vi "ABB Calc efficiency2.vi"(0 "Rated Data":T3, 1 "max wdg rise":dbl, 2 "Stator wdg":enum16{"Star", "Delta"}(ring), 3 "Stator  Phase resistance":dbl, 5 "Ambient temp":dbl, 7 "Frequency (Hz)":dbl, 9 "Efficiency Standard":enum16{"IEC 60034", "NEMA", "IEC 61972"}(ring), 11 "Specified  Power Factor":dbl[](array[numeric]), 12 "Selected Loads (% Rated)":dbl[](array[numeric]), 13 "Ohms":cluster{"Stator":dbl[], "Rotor":dbl[]}, 14 "Losses at rated voltage":T2, 15 "slip entry":T1={"Slip Source"=enum."Calculated", "Slip Entry"=[0.0, 0.0, 0.0, 0.0]}) -> (4 "Efficiency out":dbl[][](array[numeric]), 6 "Effy Temp":dbl, 8 "R at EffyT":cluster{"Stator":dbl[], "Rotor":dbl[]})   [LabVIEW 2017]
panel:
  out "mech+Iron":dbl
  # "Calculated slip"
  # "Mechanical Loss  (kW)"
  # "Iron Loss (kW)"
  # "Stator Copper Loss (kW)"
  # "Rotor Copper Loss (kW)"
  # "Stray load loss (kW)"
  # "Total loss (kW)"
  # "Load (kW)"
  # "Efficiency (%)"
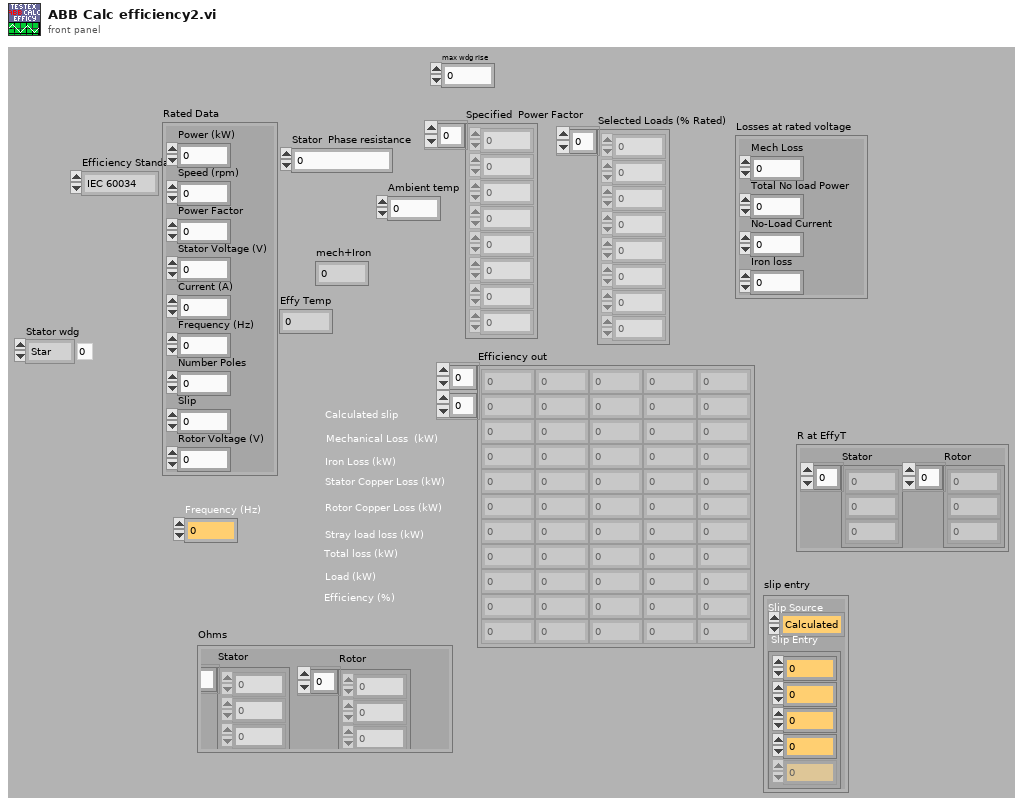
[diagram p1: front panel]
types:
  T1 = cluster{"Slip Source":enum16{"Calculated", "Entered"}, "Slip Entry":dbl[]}
  T2 = cluster{"Mech Loss":dbl, "Total No load Power":dbl, "No-Load Current":dbl, "Iron loss":dbl}
  T3 = cluster{"Power (kW)":dbl, "Speed (rpm)":dbl, "Power Factor":dbl, "Stator Voltage (V)":dbl, "Current (A)":dbl, "Frequency (Hz)":dbl, "Number Poles":dbl, "Slip":dbl, "Rotor Voltage (V)":dbl}
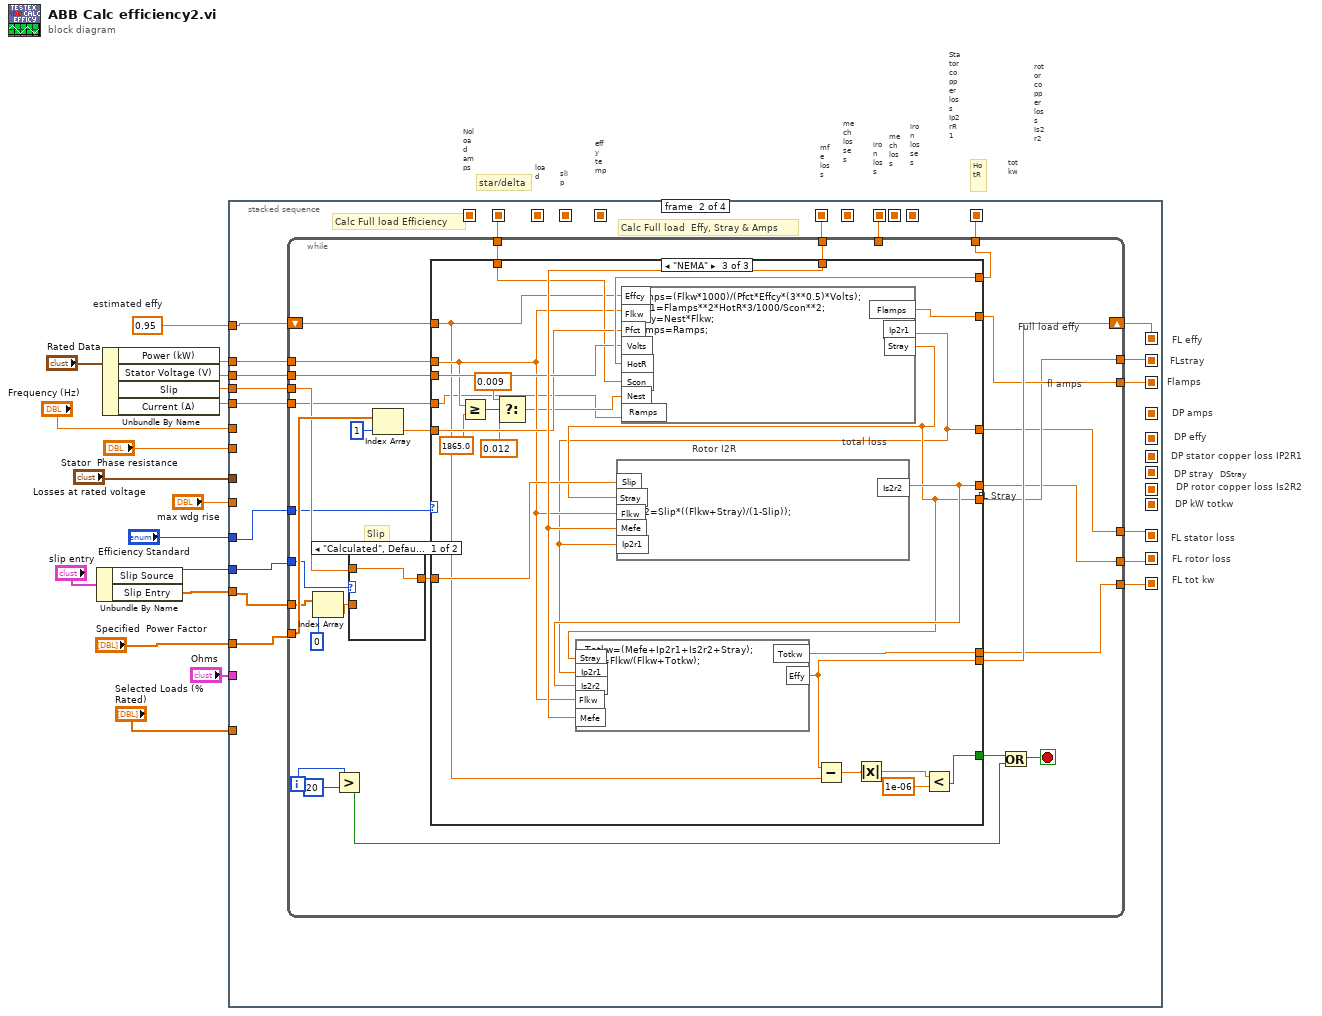
[diagram p0: block diagram]
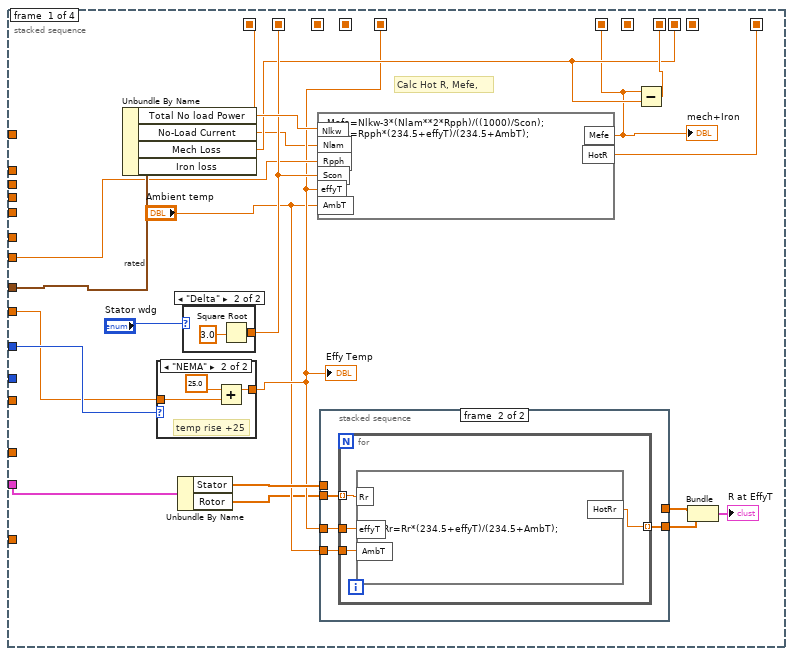
[diagram p2: hidden frame]
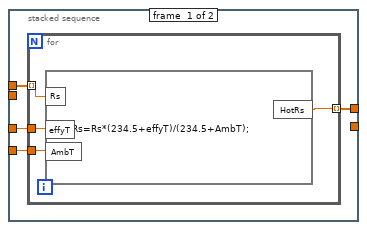
[diagram p3: hidden frame]
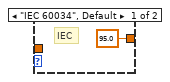
[diagram p4: hidden frame]
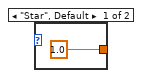
[diagram p5: hidden frame]
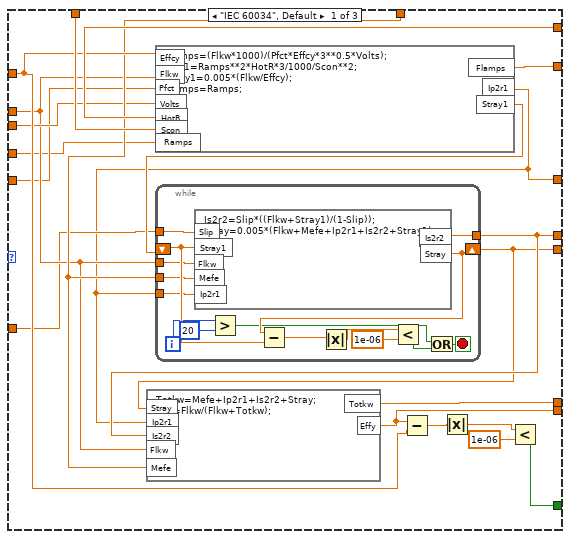
[diagram p6: hidden frame]
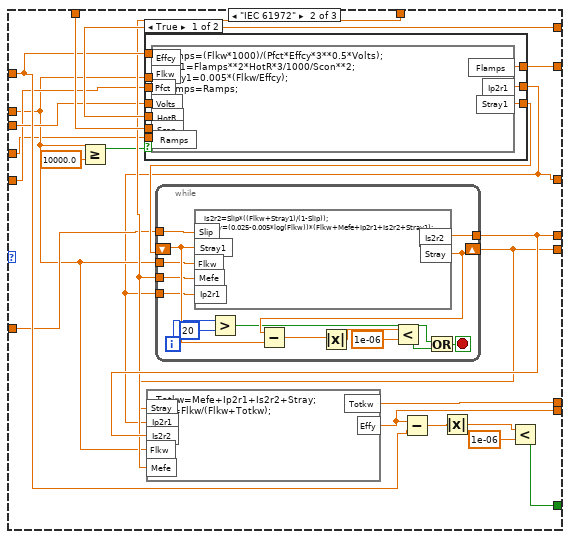
[diagram p7: hidden frame]
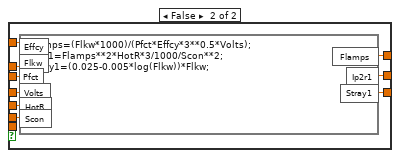
[diagram p8: hidden frame]
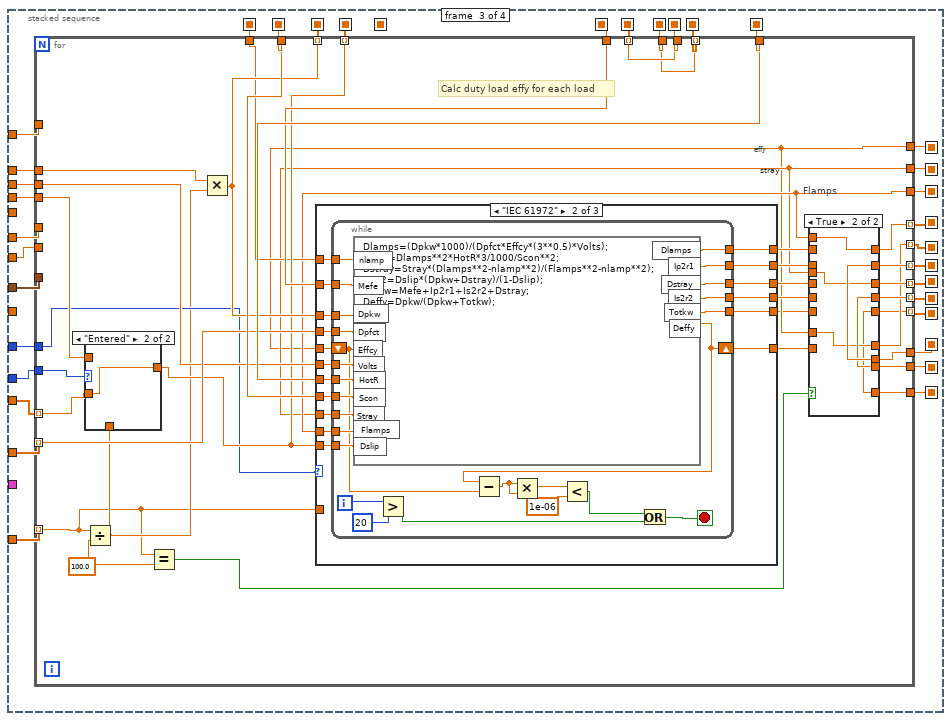
[diagram p10: hidden frame]
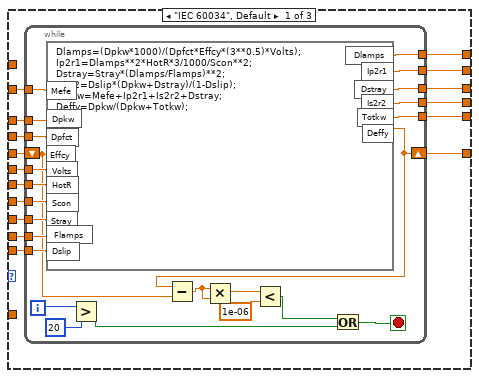
[diagram p12: hidden frame]
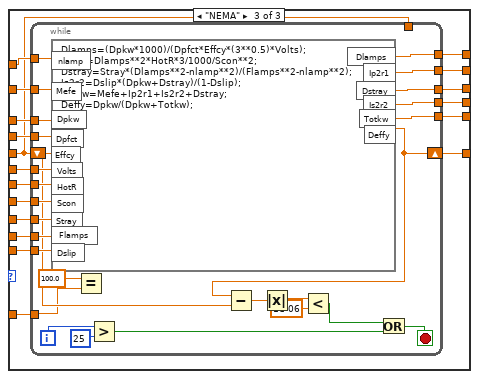
[diagram p13: hidden frame]
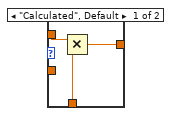
[diagram p14: hidden frame]
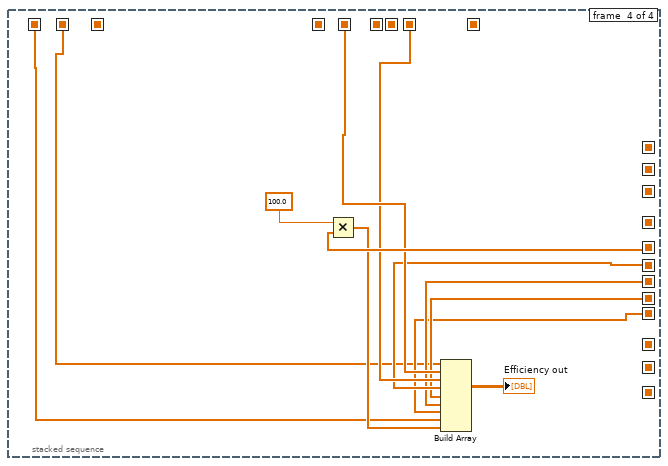
[diagram p15: hidden frame]
diagram:
  w14 = 0.95  # estimated effy
  # "FL tot kw"
  # "DP amps"
  # "FL rotor loss"
  # "FL stator loss"
  # "Noload amps"
  # "DP effy"
  # "DStray"
  # "DP kW totkw"
  # "DP rotor copper loss Is2R2"
  # "DP stray"
  # "DP stator copper loss IP2R1"
  # "Flamps"
  # "FLstray"
  # "FL effy"
  # "effy temp"
  # "mfe loss"
  # "mech losses"
  # "iron losses"
  # "iron loss"
  # "mech loss"
  # "rotor copper loss Is2r2"
  # "Stator copper loss Ip2rR1"
  # "load"
  # "tot kw"
  # "slip"
  # "star/delta"
  # "HotR"
  n1 = Unbundle By Name("slip entry") -> ("Slip Source"=w9:enum16{"Calculated", "Entered"}, "Slip Entry"=w8:dbl[])
  n2 = Unbundle By Name("Rated Data") -> ("Power (kW)"=w6:dbl, "Stator Voltage (V)"=w5:dbl, "Slip"=w4:dbl, "Current (A)"=w1:dbl)
  n3 = stacked-sequence {
    seq-local: [w31 _ _ _] -> [_ w77 w250 _]
    seq-local: [w35 _ _ _] -> [_ w78 w251 _]
    seq-local: [w33 _ _ _] -> [_ w73 w252 _]
    seq-local: [_ _ w249 _] -> [_ _ _ w449]
    seq-local: [_ _ w248 _] -> [_ _ _ w447]
    seq-local: [w30 _ _ _] -> [_ _ w247 _]
    seq-local: [_ _ w231 _] -> [_ _ _ w448]
    seq-local: [w29 _ _ _] -> [_ w79 w246 _]
    seq-local: [w26 _ _ _] -> [_ _ _ _]
    seq-local: [_ w70 _ _] -> [_ _ w240 _]
    seq-local: [_ _ w239 _] -> [_ _ _ w446]
    seq-local: [_ _ w237 _] -> [_ _ _ w444]
    seq-local: [_ _ w236 _] -> [_ _ _ w445]
    seq-local: [_ _ w238 _] -> [_ _ _ w443]
    seq-local: [_ w69 _ _] -> [_ _ w234 _]
    seq-local: [_ w68 _ _] -> [_ _ w235 _]
    seq-local: [_ _ w233 _] -> [_ _ _ w440]
    seq-local: [_ _ w232 _] -> [_ _ _ w439]
    seq-local: [_ _ w230 _] -> [_ _ _ _]
    seq-local: [w18 _ _ _] -> [_ _ w228 _]
    seq-local: [_ w64 _ _] -> [_ _ w227 _]
    seq-local: [_ w65 _ _] -> [_ _ w226 _]
    seq-local: [_ w63 _ _] -> [_ _ w225 _]
    tunnel: "Specified  Power Factor" -> [_ w72 w258 _]
    tunnel: "Selected Loads (% Rated)" -> [_ _ w257 _]
    tunnel: "Losses at rated voltage" -> [w37 _ w256 _]
    tunnel: w14 -> [_ w67 w255 _]
    tunnel: "Stator  Phase resistance" -> [w32 _ w254 _]
    tunnel: "Frequency (Hz)" -> [_ _ w253 _]
    tunnel: "Ohms" -> [w28 _ _ _]
    tunnel: w9 -> [_ w71 w245 _]
    tunnel: w8 -> [_ w62 w244 _]
    tunnel: w6 -> [_ w76 w243 _]
    tunnel: w5 -> [_ w75 w242 _]
    tunnel: w4 -> [_ w74 w241 _]
    tunnel: "Efficiency Standard" -> [w20 w66 w229 _]
    tunnel: "max wdg rise" -> [w19 _ _ _]
    tunnel: w1 -> [_ w61 _ _]
    frame #0 {
      # "Calc Hot R, Mefe,"
      # "rated"
      n4 = Unbundle By Name(w37) -> ("Total No load Power"=w36:dbl, "No-Load Current"=w18:dbl, "Mech Loss"=w30:dbl)  [unwired: 1 out]
      n5 = case shown="\"NEMA\"" w20 {
        tunnel: [95.0 w55] -> w26
        tunnel: w19 -> [_ w56]
        frame "IEC 60034", Default {
          # "IEC"
        }
        frame "NEMA" {
          # "temp rise +25"
          n6 = Add(x=25.0, y=w56) -> (x+y=w55:dbl)
        }
      }
      "Effy Temp" <- w26
      n7 = Unbundle By Name(w28) -> ("Stator"=w27:dbl[], "Rotor"=w24:dbl[])
      n8 = case shown="\"Delta\"" "Stator wdg" {
        tunnel: [1.0 w59] -> w33
        frame "Star", Default {
        }
        frame "Delta" {
          n9 = Square Root(x=3.0) -> (sqrt(x)=w59:dbl)
        }
      }
      n10 = formula code="Mefe=Nlkw-3*(Nlam**2*Rpph)/((1000)/Scon);\nHotR=Rpph*(234.5+effyT)/(234.5+AmbT);"("Nlkw"=w36, "Nlam"=w18, "Rpph"=w32, "Scon"=w33, "effyT"=w26, "AmbT"="Ambient temp") -> ("Mefe"=w29:dbl, "HotR"=w35:dbl)
      "mech+Iron" <- w29
      n11 = stacked-sequence {
        tunnel: w27 -> [w40 _]
        tunnel: w26 -> [w41 w49]
        tunnel: "Ambient temp" -> [w39 w48]
        tunnel: [w38 _] -> w23
        tunnel: w24 -> [_ w47]
        tunnel: [_ w46] -> w22
        frame #0 {
          n12 = for {
            tunnel: w41 -> [w45]
            tunnel: w40 -> [w44] mode=indexing
            tunnel: w39 -> [w43]
            tunnel: [w42] -> w38 mode=indexing
            n13 = formula code="HotRs=Rs*(234.5+effyT)/(234.5+AmbT);"("Rs"=w44, "effyT"=w45, "AmbT"=w43) -> ("HotRs"=w42:dbl)
          }
        }
        frame #1 {
          n14 = for {
            tunnel: w49 -> [w53]
            tunnel: w48 -> [w52]
            tunnel: [w51] -> w46 mode=indexing
            tunnel: w47 -> [w50] mode=indexing
            n15 = formula code="HotRr=Rr*(234.5+effyT)/(234.5+AmbT);"("Rr"=w50, "effyT"=w53, "AmbT"=w52) -> ("HotRr"=w51:dbl)
          }
        }
      }
      n16 = Subtract(x=w29, y=w30) -> (x-y=w31:dbl)
      n17 = Bundle(w23, w22) -> (→"R at EffyT":cluster{dbl[], dbl[]})  [unwired: 1 in]
    }
    frame #1 {
      # "Calc Full load  Effy, Stray & Amps"
      # "Calc Full load Efficiency"
      n18 = while {
        tunnel: w72 -> [w107]
        shift-right: [w95] -> w70
        shift-left: w67 -> [w100]
        tunnel: w73 -> [w102]
        tunnel: w78 -> [w101]
        tunnel: w77 -> [_]
        tunnel: w79 -> [w98]
        tunnel: w71 -> [w97]
        tunnel: w62 -> [w96]
        tunnel: w76 -> [w92]
        tunnel: w75 -> [w94]
        tunnel: w74 -> [w93]
        tunnel: [w91] -> w69
        tunnel: [w85] -> w68
        tunnel: w66 -> [w84]
        tunnel: [w83] -> w65
        tunnel: [w82] -> w64
        tunnel: [w81] -> w63
        tunnel: w61 -> [w80]
        i -> [w106]
        stop <- w104 stop-if-true
        # "fl amps"
        # "FL Stray"
        # "Full load effy"
        # "Slip"
        n19 = Index Array(array=w96, index=0) -> (element=w87:dbl)
        n20 = Greater?(x=w106, y=20) -> (0:w103:bool)
        n21 = case shown="\"Calculated\", Default" w97 {
          tunnel: w93 -> [w223 _]
          tunnel: [w223 w224] -> w90
          tunnel: w87 -> [_ w224]
          frame "Calculated", Default {
          }
          frame "Entered" {
          }
        }
        n22 = Index Array(array=w107, index=1) -> (element=w89:dbl)
        n23 = case shown="\"NEMA\"" w84 {
          tunnel: w102 -> [w127 w164 w214]
          tunnel: w101 -> [w126 w163 w222]
          tunnel: w100 -> [w124 w161 w202]
          tunnel: [w121 w158 w203] -> w99
          tunnel: [w119 w156 w221] -> w81
          tunnel: [w118 w155 w220] -> w83
          tunnel: w98 -> [w117 w154 w219]
          tunnel: [w116 w153 w201] -> w95
          tunnel: w94 -> [w115 w152 w218]
          tunnel: w92 -> [w114 w147 w213]
          tunnel: [w109 w151 w217] -> w91
          tunnel: w90 -> [w113 w150 w216]
          tunnel: w89 -> [w112 w149 w215]
          tunnel: [w111 w148 w207] -> w85
          tunnel: [w110 w144 w200] -> w82
          tunnel: w80 -> [w108 w143 w199]
          frame "IEC 60034", Default {
            n24 = formula code="Flamps=(Flkw*1000)/(Pfct*Effcy*3**0.5*Volts);\nIp2r1=Ramps**2*HotR*3/1000/Scon**2;\nStray1=0.005*(Flkw/Effcy);\nFlamps=Ramps;"("Effcy"=w124, "Flkw"=w114, "Pfct"=w112, "Volts"=w115, "HotR"=w126, "Scon"=w127, "Ramps"=w108) -> ("Flamps"=w109:dbl, "Ip2r1"=w110:dbl, "Stray1"=w125:dbl)
            n25 = while {
              tunnel: w113 -> [w142]
              shift-right: [w141] -> w111
              shift-left: w125 -> [w140]
              tunnel: w114 -> [w135]
              tunnel: w117 -> [w134]
              tunnel: w110 -> [w133]
              tunnel: [w132] -> w118
              i -> [w131]
              stop <- w129 stop-if-true
              n26 = formula code="Is2r2=Slip*((Flkw+Stray1)/(1-Slip));\nStray=0.005*(Flkw+Mefe+Ip2r1+Is2r2+Stray1);"("Slip"=w142, "Stray1"=w140, "Flkw"=w135, "Mefe"=w134, "Ip2r1"=w133) -> ("Is2r2"=w132:dbl, "Stray"=w141:dbl)
              n27 = Greater?(x=w131, y=20) -> (0:w128:bool)
              n28 = Subtract(x=w141, y=w140) -> (x-y=w139:dbl)
              n29 = Absolute Value(x=w139) -> (abs(x)=w138:dbl)
              n30 = Less?(x=w138, y=1e-06) -> (x < y?=w136:bool)
              n31 = Or(x=w128, y=w136) -> (x .or. y?=w129:bool)
            }
            n32 = formula code="Totkw=Mefe+Ip2r1+Is2r2+Stray;\nEffy=Flkw/(Flkw+Totkw);"("Stray"=w111, "Ip2r1"=w110, "Is2r2"=w118, "Mefe"=w117, "Flkw"=w114) -> ("Totkw"=w119:dbl, "Effy"=w116:dbl)
            n33 = Subtract(x=w116, y=w124) -> (x-y=w123:dbl)
            n34 = Absolute Value(x=w123) -> (abs(x)=w122:dbl)
            n35 = Less?(x=w122, y=1e-06) -> (x < y?=w121:bool)
          }
          frame "IEC 61972" {
            n36 = Greater Or Equal?(x=w147, y=10000.0) -> (x >= y?=w145:bool)
            n37 = case shown="True" w145 {
              tunnel: w164 -> [w174 w183]
              tunnel: w163 -> [w173 w182]
              tunnel: [w172 w181] -> w162
              tunnel: w161 -> [w171 w180]
              tunnel: [w170 w179] -> w144
              tunnel: w152 -> [w169 w178]
              tunnel: w147 -> [w168 w177]
              tunnel: [w167 w176] -> w151
              tunnel: w149 -> [w166 w175]
              tunnel: w143 -> [w165 _]
              frame True {
                n38 = formula code="Flamps=(Flkw*1000)/(Pfct*Effcy*3**0.5*Volts);\nIp2r1=Flamps**2*HotR*3/1000/Scon**2;\nStray1=0.005*(Flkw/Effcy);\nFlamps=Ramps;"("Effcy"=w171, "Flkw"=w168, "Pfct"=w166, "Volts"=w169, "HotR"=w173, "Scon"=w174, "Ramps"=w165) -> ("Flamps"=w167:dbl, "Ip2r1"=w170:dbl, "Stray1"=w172:dbl)
              }
              frame False {
                n39 = formula code="Flamps=(Flkw*1000)/(Pfct*Effcy*3**0.5*Volts);\nIp2r1=Flamps**2*HotR*3/1000/Scon**2;\nStray1=(0.025-0.005*log(Flkw))*Flkw;"("Effcy"=w180, "Flkw"=w177, "Pfct"=w175, "Volts"=w178, "HotR"=w182, "Scon"=w183) -> ("Flamps"=w176:dbl, "Ip2r1"=w179:dbl, "Stray1"=w181:dbl)
              }
            }
            n40 = while {
              tunnel: w150 -> [w198]
              shift-right: [w197] -> w148
              shift-left: w162 -> [w196]
              tunnel: w147 -> [w191]
              tunnel: w154 -> [w190]
              tunnel: w144 -> [w189]
              tunnel: [w188] -> w155
              i -> [w187]
              stop <- w185 stop-if-true
              n41 = formula code="Is2r2=Slip*((Flkw+Stray1)/(1-Slip));\nStray=(0.025-0.005*log(Flkw))*(Flkw+Mefe+Ip2r1+Is2r2+Stray1);"("Slip"=w198, "Stray1"=w196, "Flkw"=w191, "Mefe"=w190, "Ip2r1"=w189) -> ("Is2r2"=w188:dbl, "Stray"=w197:dbl)
              n42 = Greater?(x=w187, y=20) -> (0:w184:bool)
              n43 = Subtract(x=w197, y=w196) -> (x-y=w195:dbl)
              n44 = Absolute Value(x=w195) -> (abs(x)=w194:dbl)
              n45 = Less?(x=w194, y=1e-06) -> (x < y?=w192:bool)
              n46 = Or(x=w184, y=w192) -> (x .or. y?=w185:bool)
            }
            n47 = formula code="Totkw=Mefe+Ip2r1+Is2r2+Stray;\nEffy=Flkw/(Flkw+Totkw);"("Stray"=w148, "Ip2r1"=w144, "Is2r2"=w155, "Mefe"=w154, "Flkw"=w147) -> ("Totkw"=w156:dbl, "Effy"=w153:dbl)
            n48 = Subtract(x=w153, y=w161) -> (x-y=w160:dbl)
            n49 = Absolute Value(x=w160) -> (abs(x)=w159:dbl)
            n50 = Less?(x=w159, y=1e-06) -> (x < y?=w158:bool)
          }
          frame "NEMA" {
            # "Rotor I2R"
            # "total loss"
            n51 = Greater Or Equal?(x=w213, y=1865.0) -> (x >= y?=w211:bool)
            n52 = Select(t=0.009, s=w211, f=0.012) -> (s? t:f=w208:dbl)
            n53 = formula code="Flamps=(Flkw*1000)/(Pfct*Effcy*(3**0.5)*Volts);\nIp2r1=Flamps**2*HotR*3/1000/Scon**2;\nStray=Nest*Flkw;\nFlamps=Ramps;"("Effcy"=w202, "Flkw"=w213, "Pfct"=w215, "Volts"=w218, "HotR"=w222, "Scon"=w214, "Nest"=w208, "Ramps"=w199) -> ("Flamps"=w217:dbl, "Ip2r1"=w200:dbl, "Stray"=w207:dbl)
            n54 = formula code="Is2r2=Slip*((Flkw+Stray)/(1-Slip));"("Slip"=w216, "Stray"=w207, "Flkw"=w213, "Mefe"=w219, "Ip2r1"=w200) -> ("Is2r2"=w220:dbl)
            n55 = formula code="Totkw=(Mefe+Ip2r1+Is2r2+Stray);\nEffy=Flkw/(Flkw+Totkw);"("Stray"=w207, "Ip2r1"=w200, "Is2r2"=w220, "Mefe"=w219, "Flkw"=w213) -> ("Totkw"=w221:dbl, "Effy"=w201:dbl)
            n56 = Subtract(x=w201, y=w202) -> (x-y=w206:dbl)
            n57 = Absolute Value(x=w206) -> (abs(x)=w205:dbl)
            n58 = Less?(x=w205, y=1e-06) -> (x < y?=w203:bool)
          }
        }
        n59 = Or(x=w99, y=w103) -> (x .or. y?=w104:bool)
      }
    }
    frame #2 {
      n60 = for {
        tunnel: w258 -> [w290] mode=indexing
        tunnel: w257 -> [w259] mode=indexing
        tunnel: w253 -> [_]
        tunnel: w256 -> [_]
        tunnel: w255 -> [_]
        tunnel: w254 -> [_]
        tunnel: [w269] -> w249 mode=indexing
        tunnel: w252 -> [w295]
        tunnel: w251 -> [w294]
        tunnel: w250 -> [w284]
        tunnel: [w293] -> w233 mode=indexing
        tunnel: [w284] -> w248 mode=indexing
        tunnel: w247 -> [w285]
        tunnel: w246 -> [w292]
        tunnel: w245 -> [w291]
        tunnel: w244 -> [w283] mode=indexing
        tunnel: w243 -> [w289]
        tunnel: w242 -> [w288]
        tunnel: w241 -> [w287]
        tunnel: w240 -> [w263]
        tunnel: [w275] -> w239 mode=indexing
        tunnel: [w273] -> w237 mode=indexing
        tunnel: [w271] -> w236 mode=indexing
        tunnel: [w261] -> w238 mode=indexing
        tunnel: w235 -> [w264]
        tunnel: w234 -> [w267]
        tunnel: [w286] -> w232 mode=indexing
        tunnel: [w285] -> w231 mode=indexing
        tunnel: [w277] -> w230 mode=indexing
        tunnel: w229 -> [w282]
        tunnel: w228 -> [w281]
        tunnel: w227 -> [w266]
        tunnel: w226 -> [w265]
        tunnel: w225 -> [w260]
        w279 = 100.0 ("y")
        # "Flamps"
        # "stray"
        # "effy"
        # "Calc duty load effy for each load"
        n61 = Divide(x=w259, y=w279) -> (x/y=w280:dbl)
        n62 = case shown="\"Entered\"" w291 {
          tunnel: w287 -> [w437 _]
          tunnel: w280 -> [w436 _]
          tunnel: [w435 w438] -> w286
          tunnel: w283 -> [_ w438]
          frame "Calculated", Default {
            n63 = Multiply(x=w437, y=w436) -> (x*y=w435:dbl)
          }
          frame "Entered" {
          }
        }
        n64 = Equal?(x=w259, y=w279) -> (x = y?=w268:bool)
        n65 = Multiply(x=w289, y=w280) -> (x*y=w293:dbl)
        n66 = case shown="\"IEC 61972\"" w282 {
          tunnel: w295 -> [w323 w364 w407]
          tunnel: w294 -> [w322 w363 w406]
          tunnel: [w321 w362 w405] -> w270
          tunnel: w293 -> [w320 w361 w404]
          tunnel: w292 -> [w319 w360 w403]
          tunnel: w290 -> [w318 w359 w402]
          tunnel: w288 -> [w317 w358 w401]
          tunnel: [w316 w357 w400] -> w276
          tunnel: [w315 w356 w390] -> w274
          tunnel: [w314 w355 w399] -> w272
          tunnel: [w313 w354 w398] -> w262
          tunnel: w263 -> [w312 w353 w391]
          tunnel: w264 -> [w311 w352 w397]
          tunnel: w267 -> [w310 w351 w396]
          tunnel: w286 -> [w309 w350 w395]
          tunnel: [w308 w349 w394] -> w278
          tunnel: w281 -> [_ w348 w393]
          tunnel: w259 -> [_ _ w392]
          frame "IEC 60034", Default {
            n67 = while {
              tunnel: w320 -> [w345]
              tunnel: w318 -> [w344]
              tunnel: w317 -> [w343]
              tunnel: w322 -> [w341]
              tunnel: w323 -> [w340]
              tunnel: w311 -> [w339]
              tunnel: w310 -> [w338]
              tunnel: w309 -> [w337]
              tunnel: w319 -> [w336]
              shift-right: [w329] -> w321
              shift-left: w312 -> [w335]
              tunnel: [w328] -> w316
              tunnel: [w327] -> w315
              tunnel: [w326] -> w314
              tunnel: [w325] -> w313
              tunnel: [w324] -> w308
              i -> [w347]
              stop <- w331 stop-if-true
              n68 = formula code="Dlamps=(Dpkw*1000)/(Dpfct*Effcy*(3**0.5)*Volts);\nIp2r1=Dlamps**2*HotR*3/1000/Scon**2;\nDstray=Stray*(Dlamps/Flamps)**2;\nIs2r2=Dslip*(Dpkw+Dstray)/(1-Dslip);\nTotkw=Mefe+Ip2r1+Is2r2+Dstray;\nDeffy=Dpkw/(Dpkw+Totkw);"("Dpkw"=w345, "Dpfct"=w344, "Effcy"=w335, "Volts"=w343, "HotR"=w341, "Scon"=w340, "Stray"=w339, "Flamps"=w338, "Dslip"=w337, "Mefe"=w336) -> ("Dlamps"=w324:dbl, "Ip2r1"=w328:dbl, "Dstray"=w327:dbl, "Is2r2"=w326:dbl, "Totkw"=w325:dbl, "Deffy"=w329:dbl)
              n69 = Greater?(x=w347, y=20) -> (0:w342:bool)
              n70 = Subtract(x=w329, y=w335) -> (x-y=w334:dbl)
              n71 = Multiply(x=w334, y=w334) -> (x*y=w333:dbl)
              n72 = Less?(x=w333, y=1e-06) -> (x < y?=w330:bool)
              n73 = Or(x=w330, y=w342) -> (x .or. y?=w331:bool)
            }
          }
          frame "IEC 61972" {
            n74 = while {
              tunnel: w361 -> [w387]
              tunnel: w359 -> [w386]
              tunnel: w358 -> [w385]
              tunnel: w363 -> [w383]
              tunnel: w364 -> [w382]
              tunnel: w352 -> [w381]
              tunnel: w351 -> [w380]
              tunnel: w350 -> [w379]
              tunnel: w360 -> [w378]
              shift-right: [w371] -> w362
              shift-left: w353 -> [w377]
              tunnel: [w370] -> w357
              tunnel: [w369] -> w356
              tunnel: [w368] -> w355
              tunnel: [w367] -> w354
              tunnel: [w366] -> w349
              tunnel: w348 -> [w365]
              i -> [w389]
              stop <- w373 stop-if-true
              n75 = formula code="Dlamps=(Dpkw*1000)/(Dpfct*Effcy*(3**0.5)*Volts);\nIp2r1=Dlamps**2*HotR*3/1000/Scon**2;\nDstray=Stray*(Dlamps**2-nlamp**2)/(Flamps**2-nlamp**2);\nIs2r2=Dslip*(Dpkw+Dstray)/(1-Dslip);\nTotkw=Mefe+Ip2r1+Is2r2+Dstray;\nDeffy=Dpkw/(Dpkw+Totkw);"("Dpkw"=w387, "Dpfct"=w386, "Effcy"=w377, "Volts"=w385, "HotR"=w383, "Scon"=w382, "Stray"=w381, "Flamps"=w380, "Dslip"=w379, "Mefe"=w378, "nlamp"=w365) -> ("Dlamps"=w366:dbl, "Ip2r1"=w370:dbl, "Dstray"=w369:dbl, "Is2r2"=w368:dbl, "Totkw"=w367:dbl, "Deffy"=w371:dbl)
              n76 = Greater?(x=w389, y=20) -> (0:w384:bool)
              n77 = Subtract(x=w371, y=w377) -> (x-y=w376:dbl)
              n78 = Multiply(x=w376, y=w376) -> (x*y=w375:dbl)
              n79 = Less?(x=w375, y=1e-06) -> (x < y?=w372:bool)
              n80 = Or(x=w372, y=w384) -> (x .or. y?=w373:bool)
            }
          }
          frame "NEMA" {
            n81 = while {
              tunnel: w407 -> [w434]
              tunnel: w406 -> [w433]
              tunnel: w404 -> [w432]
              tunnel: w403 -> [w431]
              tunnel: w402 -> [w430]
              tunnel: w401 -> [w429]
              tunnel: [w428] -> w400
              tunnel: [w427] -> w399
              tunnel: [w426] -> w398
              tunnel: w397 -> [w425]
              tunnel: w396 -> [w424]
              tunnel: w395 -> [w423]
              tunnel: [w422] -> w394
              tunnel: w393 -> [w421]
              shift-right: [w420] -> w405
              shift-left: w391 -> [w419]
              tunnel: w392 -> [w410]
              tunnel: w391 -> [_]
              tunnel: [w408] -> w390
              i -> [w413]
              stop <- w414 stop-if-true
              n82 = formula code="Dlamps=(Dpkw*1000)/(Dpfct*Effcy*(3**0.5)*Volts);\nIp2r1=Dlamps**2*HotR*3/1000/Scon**2;\nDstray=Stray*(Dlamps**2-nlamp**2)/(Flamps**2-nlamp**2);\nIs2r2=Dslip*(Dpkw+Dstray)/(1-Dslip);\nTotkw=Mefe+Ip2r1+Is2r2+Dstray;\nDeffy=Dpkw/(Dpkw+Totkw);"("Dpkw"=w432, "Dpfct"=w430, "Effcy"=w419, "Volts"=w429, "HotR"=w433, "Scon"=w434, "Stray"=w425, "Flamps"=w424, "Dslip"=w423, "Mefe"=w431, "nlamp"=w421) -> ("Dlamps"=w422:dbl, "Ip2r1"=w428:dbl, "Dstray"=w408:dbl, "Is2r2"=w427:dbl, "Totkw"=w426:dbl, "Deffy"=w420:dbl)
              n83 = Equal?(x=100.0, y=w410) -> ()  [unwired: 1 out]
              n84 = Greater?(x=w413, y=25) -> (0:w411:bool)
              n85 = Subtract(x=w420, y=w419) -> (x-y=w418:dbl)
              n86 = Absolute Value(x=w418) -> (abs(x)=w417:dbl)
              n87 = Less?(x=w417, y=1e-06) -> (x < y?=w415:bool)
              n88 = Or(x=w415, y=w411) -> (x .or. y?=w414:bool)
            }
          }
        }
        n89 = case shown="True" w268 {
          tunnel: w278 -> [w301 _]
          tunnel: [w301 w307] -> w277
          tunnel: w276 -> [w300 _]
          tunnel: [w300 w306] -> w275
          tunnel: w274 -> [w299 _]
          tunnel: [w299 w304] -> w273
          tunnel: w272 -> [w298 _]
          tunnel: [w298 w305] -> w271
          tunnel: w270 -> [w297 _]
          tunnel: [w297 w303] -> w269
          tunnel: w267 -> [_ w307]
          tunnel: w266 -> [_ w306]
          tunnel: w265 -> [_ w305]
          tunnel: w264 -> [_ w304]
          tunnel: w263 -> [_ w303]
          tunnel: w262 -> [w296 _]
          tunnel: [w296 w302] -> w261
          tunnel: w260 -> [_ w302]
          frame False {
          }
          frame True {
          }
        }
      }
    }
    frame #3 {
      n90 = Multiply(x=100.0 ("estimated effy"), y=w449) -> (x*y=w442:dbl[])
      n91 = Build Array(w439, w448, w447, w446, w445, w444, w443, w440, w442) -> (→"Efficiency out":dbl[][])
    }
  }
